vi "Image Processing Handler Create.vi"(4 "tx data queue":refnum<queue>, 5 "Camera? (F)":bool, 6 "data queue":refnum<queue>, 7 "Video Processor":refnum<class "Video Processor.lvclass">, 8 "error in (no error)":errorcluster, 11 "Image Processing Handler in":refnum<class "Headless Image Processing Handler.lvclass">) -> (0 "error out":errorcluster, 3 "Image Processing Handler out":refnum<class "Headless Image Processing Handler.lvclass">)   [LabVIEW 2018, in "Headless Image Processing Handler.lvclass"]
uses:
  Headless Image Processing Handler.lvclass
  Message/Message.lvclass
  Video Processor/Video Processor.lvclass
  Headless Image Processing Handler.lvclass/Headless Image Processing Handler.ctl
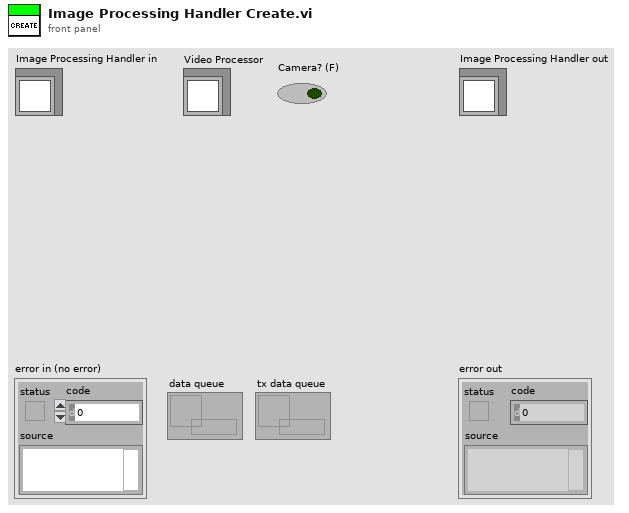
[diagram p1: front panel]
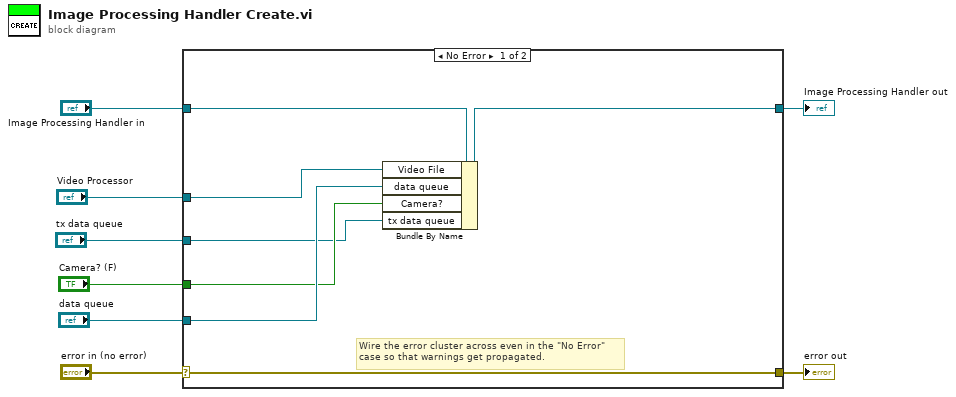
[diagram p0: block diagram]
diagram:
  n1 = case shown="No Error" "error in (no error)" {
    selector: "error in (no error)" -> [w15 w17]
    tunnel: [w15 w17] -> w7
    tunnel: [w13 w16] -> w5
    tunnel: "Image Processing Handler in" -> [w14 w16]
    tunnel: "data queue" -> [w12 _]
    tunnel: "Video Processor" -> [w11 _]
    tunnel: "Camera? (F)" -> [w10 _]
    tunnel: "tx data queue" -> [w9 _]
    frame No Error {
      # "Wire the error cluster across even in the \"No Error\"\ncase so that warnings get propagated."
      n2 = Bundle By Name(cluster=w14, "Video File"=w11, "data queue"=w12, "Camera?"=w10, "tx data queue"=w9) -> (w13:refnum<class "Headless Image Processing Handler.lvclass">)
    }
    frame Error {
    }
  }
  "error out" <- w7
  "Image Processing Handler out" <- w5
